vi "Compose JSON String (LV).vi"(8 "error in (no error)":errorcluster, 11 "Value":variant) -> (0 "error out":errorcluster, 3 "String":string)   [LabVIEW 2015, in "JSON.lvlib"]
uses:
  JSON.lvlib
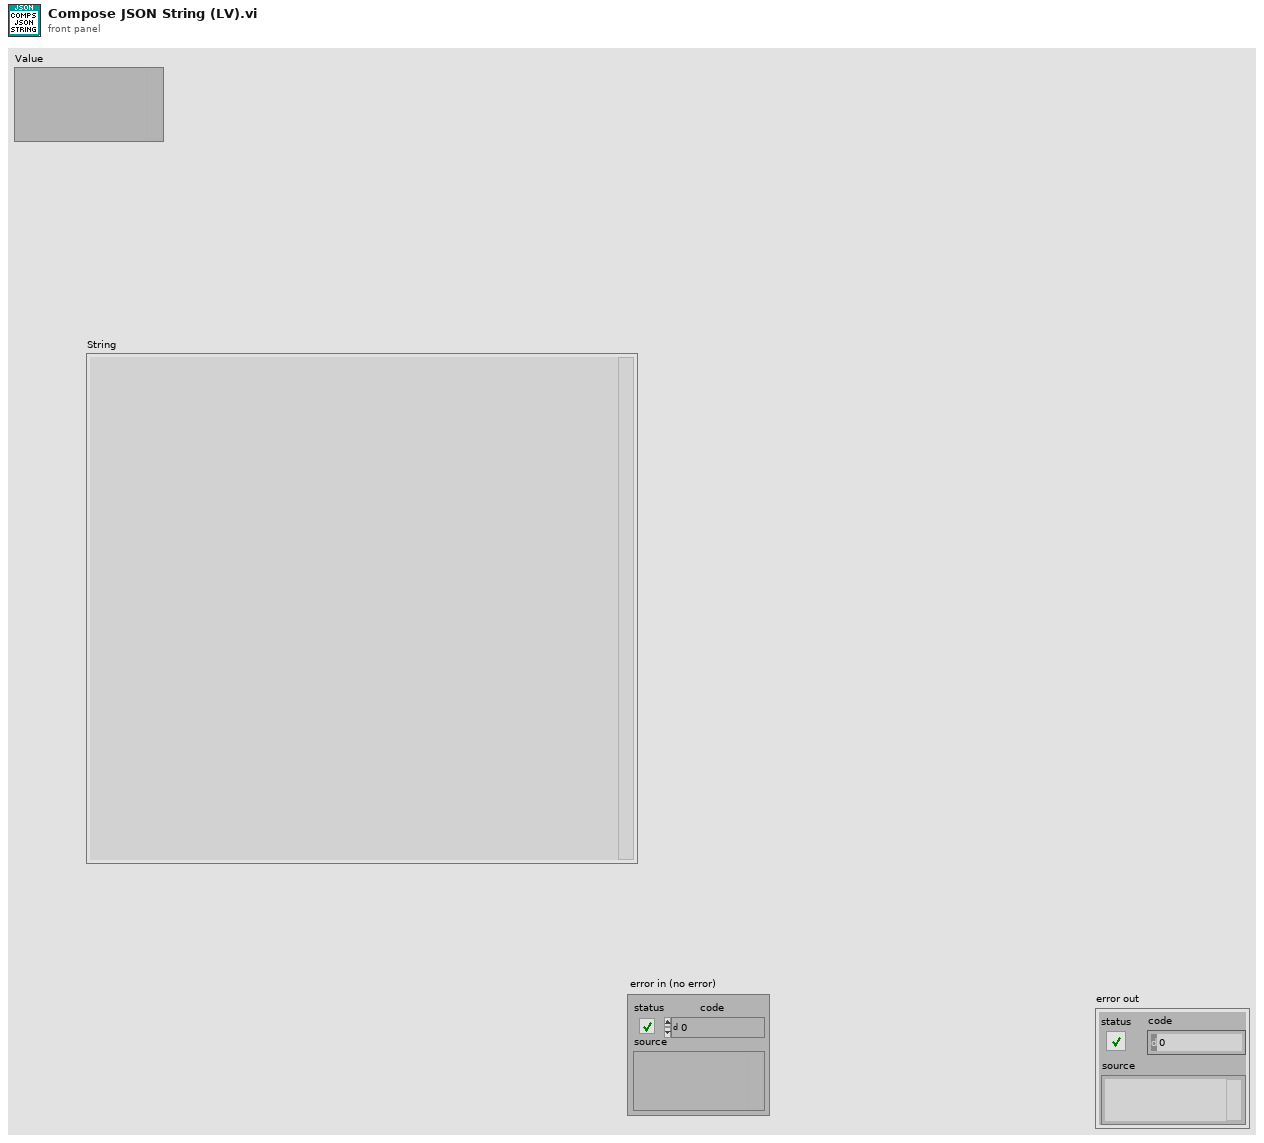
[diagram p1: front panel]
types:
  T1 = typedef "JSON.lvlib/JSON Value.ctl" = cluster{"\\type":enum16{"Object", "Array", "String", "Number", "Boolean", "Null"}, "ÿýÿýÿýÿýÿýÿþÿýÿýÿý#JSON.lvlib:JSON Name-Value Pair.ctlÿýÿýÿýÿýÿýÿþÿýÿýÿýJSON.lvlib:JSON Value.ctl":variant}
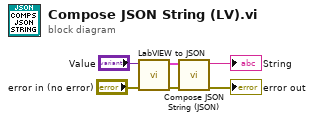
[diagram p0: block diagram]
diagram:
  n1 = call "LabVIEW to JSON.vi"("error in (no error)"="error in (no error)", "LV Value"="Value") -> ("error out"=w5:errorcluster, "JSON Value"=w6:T1)  [unwired: 8 in]
  n2 = call "Compose JSON String (JSON).vi"("error in (no error)"=w5, "Value"=w6) -> ("error out"=→"error out":errorcluster, "String"=→"String":string)  [unwired: 8 in]
